vi "pattern maker.vi"(0 "intensity graph in":dbl[][](graph), 2 "Z Scale.Range:Maximum":dbl format="%#_13g", 3 "Y Scale.Range:Maximum":dbl format="%#_13g") -> (6 "Intensity graph out":dbl[][](graph))   [LabVIEW 2016]
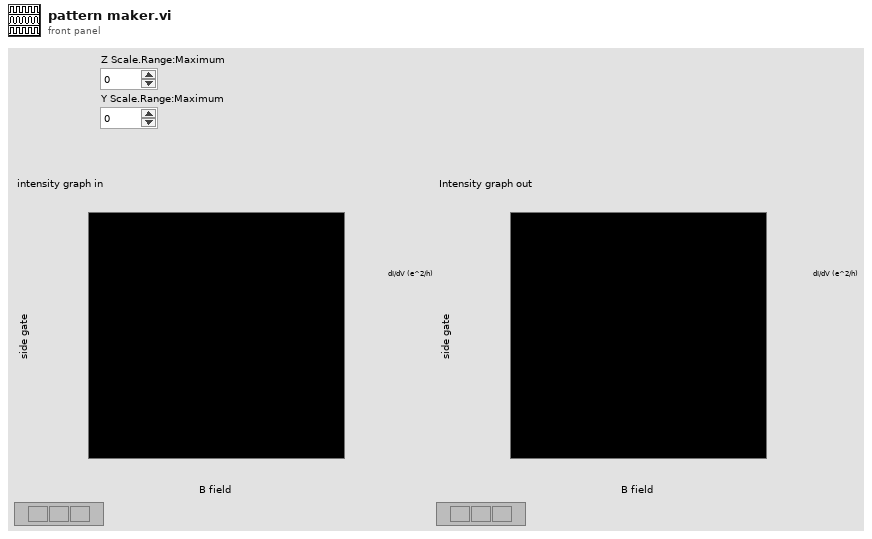
[diagram p1: front panel]
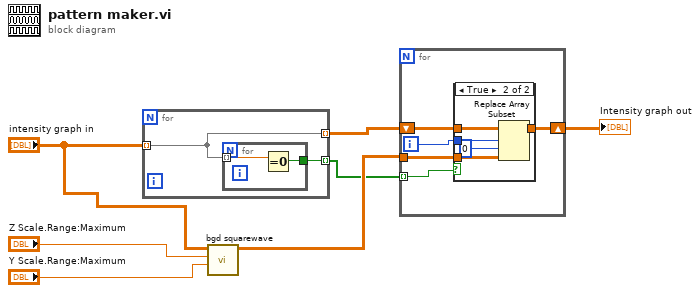
[diagram p0: block diagram]
diagram:
  n1 = for {
    tunnel: [w8] -> w7 mode=indexing
    tunnel: [w9] -> w2 mode=indexing
    tunnel: "intensity graph in" -> [w8] mode=indexing
    n2 = for {
      tunnel: [w11] -> w9
      tunnel: w8 -> [w10] mode=indexing
      n3 = Equal To 0?(x=w10) -> (x = 0?=w11:bool)
    }
  }
  n4 = call "bgd squarewave.vi"("YScale.Maximum"="Y Scale.Range:Maximum", "ZScale.Maximum"="Z Scale.Range:Maximum", "Cond. Intens. 2"="intensity graph in") -> ("square wave"=w4:dbl[][])  [unwired: 8 in]
  n5 = for {
    tunnel: w2 -> [w12] mode=indexing
    shift-right: [w14] -> w3
    shift-left: w7 -> [w15]
    tunnel: w4 -> [w13]
    i -> [w16]
    n6 = case shown="True" w12 {
      tunnel: w16 -> [_ w20]
      tunnel: w15 -> [w17 w22]
      tunnel: [w17 w21] -> w14
      tunnel: w13 -> [_ w19]
      frame False {
      }
      frame True {
        n7 = Replace Array Subset(array=w22, new element=w19, index (row)=w20, index (col)=0 ("disabled index (col)")) -> (w21:dbl[][])
      }
    }
  }
  "Intensity graph out" <- w3
